vi "PicoScope2000aExampleRapidBlockBulkMSO.vi"() -> ()   [LabVIEW 2016]
uses:
  <vilib>/Waveform/DWDTOps.llb/DWDT Analog to Digital.vi
panel:
  in  "Rapid Block Acquisition Settings":T1={"preTriggerSamples"=0, "postTriggerSamples"=1000, "timebase"=2, "Down-Sample Mode"=0, "Down Sample Ratio"=2, "Oversample"=1, "Number of Captures"=10} {"Down-Sample Mode" items=["None"=0, "Aggregate"=1, "Decimate"=2, "Average"=4]; "postTriggerSamples" format="%.6p"; "preTriggerSamples" format="%.6p"}
  out "overflow (binary)":i16 format="%06b"
  out "Port 0 Digital Waveform Graph":digitalwaveform(graph)
  in  "Port 0 Settings":cluster{"Enabled":bool, "Logic Level":i16}={"Enabled"=FALSE, "Logic Level"=9830} {"Logic Level" items=["1.5V TTL"=9830, "2.5V CMOS"=16383]}
  in  "Channel A Settings":T2={"Enabled"=TRUE, "Coupling"=1, "Range"=6, "Analogue Offset"=0.0} {"Range" items=["20 mV"=1, "50 mV"=2, "100 mV"=3, "200 mV"=4, "500 mV"=5, "1 V"=6, "2 V"=7, "5 V"=8, "10 V"=9, "20 V"=10]; "Coupling" items=["AC", "DC"]}
  out "Properties Panel":T3 {"Max Total Capture Time Available (sec)" format="%.3p"; "Sample Frequency" format="%.3p"; "Sample Internal" format="%.3p"; "Max Samples Available" format="%.3p"; "Total Capture Time (sec)" format="%.3p"}
  in  "Trigger Settings":T4={"Trigger Enabled"=FALSE, "Trigger Source"=enum."Channel A", "Trigger Threshold (Volts)"=0.0, "Trigger Direction"=2, "Trigger Delay (samples)"=0, "Auto Trigger Time (ms)"=1000} {"Trigger Direction" items=["Rising"=2, "Falling"=3]}
  out "Capture Complete":bool=TRUE
  in  "Run":bool
  out "Channel A":T5(graph)
  in  "Capture Index":u32=5
  in  "stop":bool
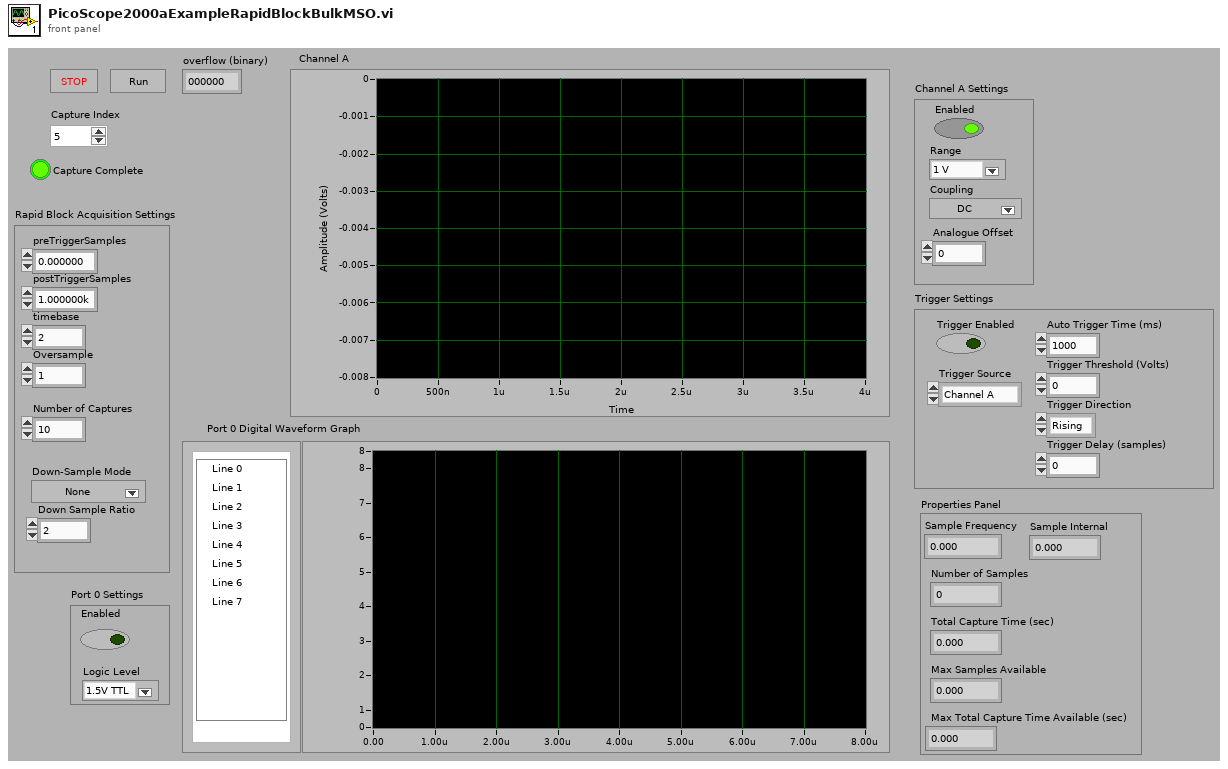
[diagram p1: front panel]
types:
  T1 = cluster{"preTriggerSamples":u32, "postTriggerSamples":u32, "timebase":u32, "Down-Sample Mode":i32, "Down Sample Ratio":u32, "Oversample":i16, "Number of Captures":u32}
  T2 = cluster{"Enabled":bool, "Coupling":i16, "Range":u16, "Analogue Offset":sgl}
  T3 = cluster{"Sample Frequency":sgl, "Sample Internal":sgl, "Max Samples Available":i32, "Number of Samples":u32, "Total Capture Time (sec) ":sgl, "Max Total Capture Time Available (sec)":sgl}
  T4 = cluster{"Trigger Enabled":bool, "Trigger Source":enum16{"Channel A", "Channel B", "Channel C", "Channel D", "Ext."}, "Trigger Threshold (Volts)":dbl, "Trigger Direction":u16, "Trigger Delay (samples)":u32, "Auto Trigger Time (ms)":i16}
  T5 = cluster{i32, "Sample Internal":sgl, "Data (Volts)":dbl[]}
  T6 = cluster{"Driver Version":string, "USB Version":string, "Hardware":string, "Variant":string, "Batch and Serial":string, "Cal Date":string, "Kernel Version":string, "Digital HW Version":string, "Analogue HW Version":string, "Firmware 1":string, "Firmware 2":string, "MSO":bool, "Number of Channels":i16}
  T7 = cluster{"preTriggerSamples":u32, "postTriggerSamples":u32, "timebase":u32, "Oversample":i16, "Down-Sample Mode":i32, "Down Sample Ratio":u32}
  T8 = cluster{i32, "Sample Internal":sgl, "Data":dbl[]}
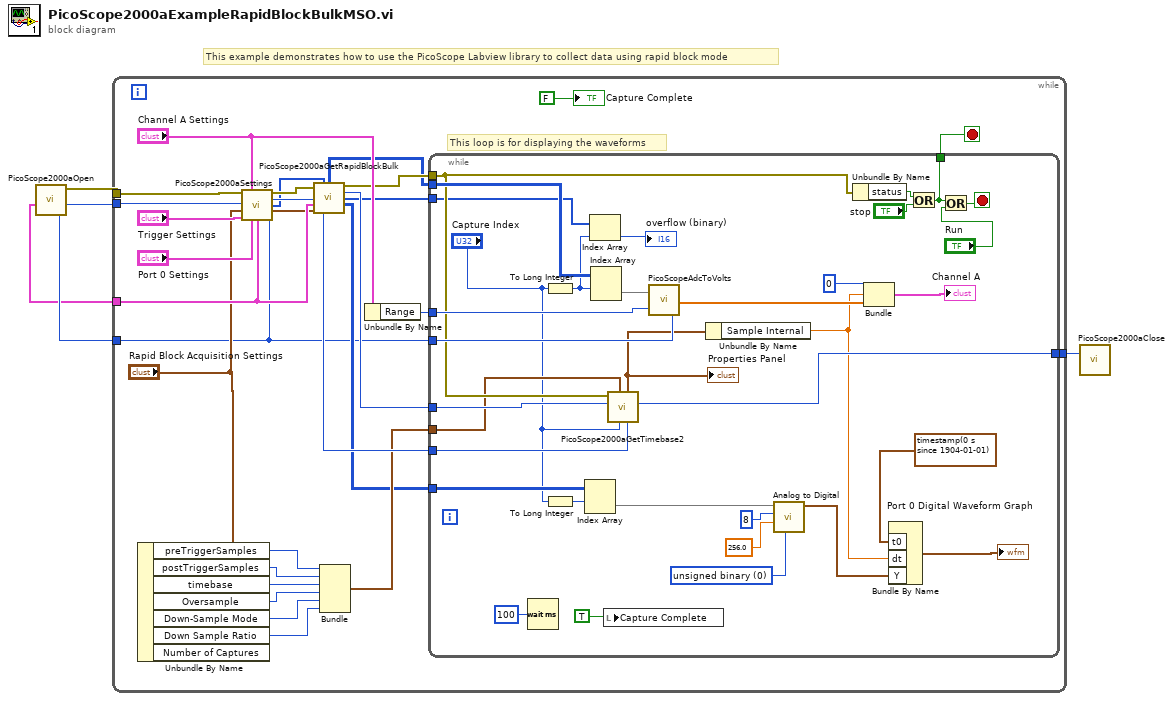
[diagram p0: block diagram]
diagram:
  # "This example demonstrates how to use the PicoScope Labview library to collect data using rapid block mode"
  n1 = call "PicoScope2000aOpen.vi"() -> ("Max Adc value"=w3:i16, "handle"=w4:i16, "error out"=w5:errorcluster, "Device Info"=w1:T6)  [unwired: 4 in]
  n2 = while {
    tunnel: w4 -> [w30]
    tunnel: w5 -> [w31]
    tunnel: w3 -> [w6]
    tunnel: [w27] -> w2
    tunnel: w1 -> [w20]
    stop <- w33 stop-if-true
    # "This loop is for displaying the waveforms"
    n3 = Unbundle By Name("Rapid Block Acquisition Settings") -> ("preTriggerSamples"=w18:u32, "postTriggerSamples"=w17:u32, "timebase"=w16:u32, "Oversample"=w15:i16, "Down-Sample Mode"=w14:i32, "Down Sample Ratio"=w12:u32)  [unwired: 1 out]
    n4 = call "PicoScope2000aSettings.vi"("error in"=w31, "Channel A Settings"="Channel A Settings", "handle in"=w30, "Trigger Settings"="Trigger Settings", "Port 0 Settings"="Port 0 Settings", "Device Info"=w20, "Max_adc"=w6) -> ("error out"=w23:errorcluster, "handle out"=w25:i16, "Enabled Array"=w9:i16[])  [unwired: 6 in]
    n5 = call "PicoScope2000aGetRapidBlockBulk.vi"("error in"=w23, "enabled array"=w9, "handle in"=w25, "Device Info"=w20, "Rapid Block Acquisition Settings"="Rapid Block Acquisition Settings") -> ("Channel A Buffer"=w22:i16[][], "error out"=w24:errorcluster, "handle out"=w21:i16, "overflow (binary)"=w8:i16[], "Port 0"=w11:i16[][], "Num samples"=w19:u32)  [unwired: 1 in, 4 out]
    n6 = Bundle("preTriggerSamples"=w18, "postTriggerSamples"=w17, "timebase"=w16, "Oversample"=w15, "Down-Sample Mode"=w14, "Down Sample Ratio"=w12) -> (w13:T7)  [unwired: 1 in]
    n7 = Unbundle By Name("Channel A Settings") -> ("Range"=w29:u16)
    n8 = while {
      tunnel: [w66] -> w33
      tunnel: w22 -> [w60]
      tunnel: w24 -> [w56]
      tunnel: w6 -> [w59]
      tunnel: w29 -> [w57]
      tunnel: w21 -> [w55]
      tunnel: [w54] -> w27
      tunnel: w19 -> [w53]
      tunnel: w13 -> [w52]
      tunnel: w11 -> [w43]
      tunnel: w8 -> [w35]
      stop <- w65 stop-if-true
      w45 = u16 0 items=["unsigned binary", "offset binary", "2's complement"] ("data format (offset binary)")
      n9 = Wait (ms)(milliseconds to wait=u32 100) -> ()  [unwired: 1 out]
      n10 = To Long Integer(number="Capture Index") -> (32bit integer=w36:i32)
      n11 = To Long Integer(number="Capture Index") -> (32bit integer=w42:i32)
      n12 = Index Array(array=w43, index (row)=w42) -> (element=w44:i16[])  [unwired: 1 in]
      n13 = Index Array(array=w35, index=w36) -> (element=→"overflow (binary)":i16)
      n14 = Index Array(array=w60, index (row)=w36) -> (element=w58:i16[])  [unwired: 1 in]
      n15 = local write "Capture Complete"(TRUE ("Capture Complete")) -> ()
      n16 = call "PicoScope2000aGetTimebase2.vi"("Number of Samples"=w53, "Memory Segment"="Capture Index", "Acquisition Settings"=w52, "handle in"=w55, "error in (no error)"=w56) -> ("handle out"=w54:i16, "Properties Panel"=w48:T3)  [unwired: 4 in, 1 out]
      "Properties Panel" <- w48
      n17 = call "PicoScopeAdcToVolts.vi"("Max_adc"=w59, "Range Index"=w57, "Data"=w58) -> ("Data"=w50:dbl[])
      n18 = Unbundle By Name(w48) -> ("Sample Internal"=w40:sgl)
      n19 = call-poly <vilib>:"Analog to Digital.vi"("data format (offset binary)"=w45, "full-scale range (pk-pk)"=256.0, "resolution (16 bit)"=8, "analog waveform"=w44) -> ("digital waveform"=w39:digitalwaveform)  [unwired: 4 in, 3 out]
      n20 = Unbundle By Name(w56) -> ("status"=w61:bool)
      n21 = Bundle(0, "Sample Internal"=w40, "Data"=w50) -> (→"Channel A":T8)  [unwired: 1 in]
      n22 = Bundle By Name("t0"=timestamp(0 s since 1904-01-01), "dt"=w40, "Y"=w39) -> (→"Port 0 Digital Waveform Graph":digitalwaveform)  [unwired: 1 in]
      n23 = Or(x=w61, y="stop") -> (x .or. y?=w66:bool)
      n24 = Or(x=w66, y="Run") -> (x .or. y?=w65:bool)
    }
    "Capture Complete" <- FALSE ("Capture Complete")
  }
  n25 = call "PicoScope2000aClose.vi"("handle"=w2) -> ()
